vi "ReadAlarms.vi"(8 "ErrorIn":errorcluster, 11 "IActionIn":refnum<class "IAction.lvclass">) -> (0 "ErrorOut":errorcluster, 2 "Alarms":refnum<class "IAlarm.lvclass">[](array[class]), 3 "IActionOut":refnum<class "IAction.lvclass">)   [LabVIEW 2019]
uses:
  IAction.lvclass
  Alarm/IAlarm.lvclass
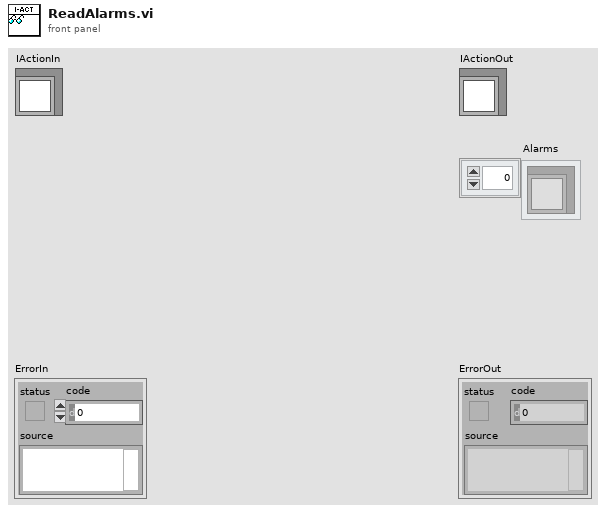
[diagram p1: front panel]
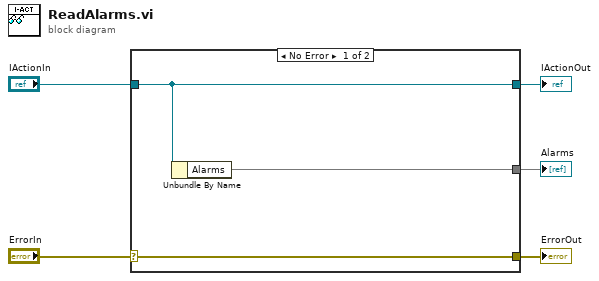
[diagram p0: block diagram]
diagram:
  n1 = case shown="No Error" "ErrorIn" {
    selector: "ErrorIn" -> [w8 w9]
    tunnel: [w8 w9] -> w4
    tunnel: [w7 w10] -> w2
    tunnel: "IActionIn" -> [w7 w10]
    tunnel: [w6 _] -> w1
    frame No Error {
      n2 = Unbundle By Name(w7) -> ("Alarms"=w6)
    }
    frame Error {
    }
  }
  "ErrorOut" <- w4
  "IActionOut" <- w2
  "Alarms" <- w1
